vi "ProgramControlTiming.vi"(0 "Front Panel Controls in":T1, 5 "Time Elapsed":dbl) -> (14 "Front Panel Controls out":T1)   [LabVIEW 2019, in "Universal Robot.lvclass"]
uses:
  Universal Robot.lvclass
  ProgramControlFPControls.ctl
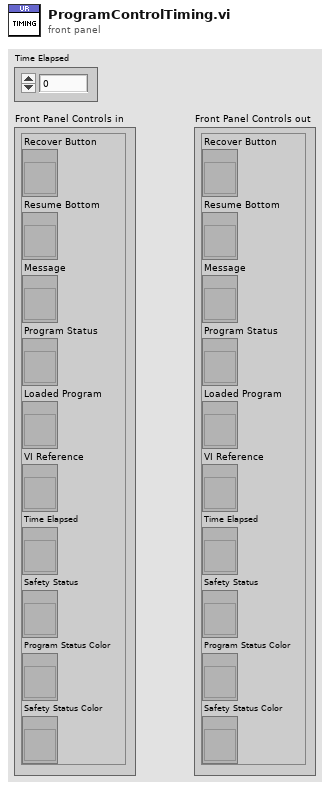
[diagram p1: front panel]
types:
  T1 = typedef "Universal Robot.lvclass/ProgramControlFPControls.ctl" = cluster{"Recover Button":refnum<vi>, "Resume Bottom":refnum<vi>, "Message":refnum<vi>, "Program Status":refnum<vi>, "Loaded Program":refnum<vi>, "VI Reference":refnum<vi>, "Time Elapsed":refnum<vi>, "Safety Status":refnum<vi>, "Program Status Color":refnum<vi>, "Safety Status Color":refnum<vi>}
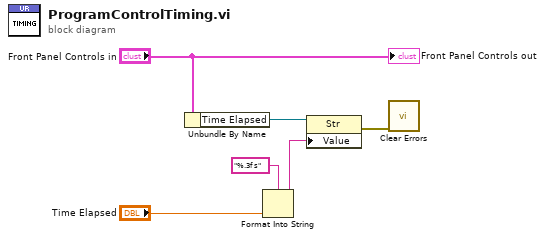
[diagram p0: block diagram]
diagram:
  n1 = Unbundle By Name("Front Panel Controls in") -> ("Time Elapsed"=w5:refnum<vi>)
  n2 = Format Into String(format string="%.3f s", "Time Elapsed") -> (resulting string=w1:string)  [unwired: 2 in, 1 out]
  n3 = property class="Str"(reference=w5, "Value"=w1) -> (error out=w4:errorcluster)  [unwired: 1 in, 1 out]
  n4 = call <vilib>:"Clear Errors.vi"("error in (no error)"=w4) -> ()  [unwired: 5 in, 2 out]
  "Front Panel Controls out" <- "Front Panel Controls in"
